vi "CodeBlockSegment.vi"(3 "error in (no error)":errorcluster caption="错误输入（无错误）", 4 "crc_data":dbl[](array[numeric]), 5 "appended path":path) -> (0 "error out":errorcluster caption="错误输出", 1 "Array":dbl[][](array[numeric]), 2 "Cluster":T1)   [LabVIEW 2015]
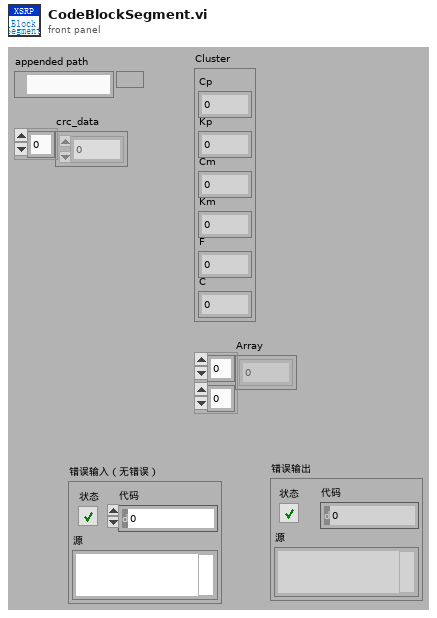
[diagram p1: front panel]
types:
  T1 = cluster{"Cp":dbl, "Kp":dbl, "Cm":dbl, "Km":dbl, "F":dbl, "C":dbl}
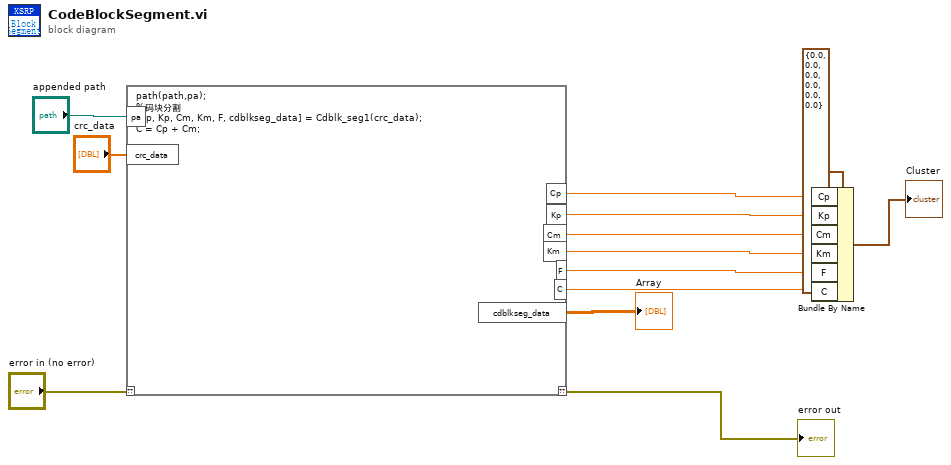
[diagram p0: block diagram]
diagram:
  n1 = script code="path(path,pa);\n%码块分割\n[Cp, Kp, Cm, Km, F, cdblkseg_data] = Cdblk_seg1(crc_data);\nC = Cp + Cm;"("??"="error in (no error)", "pa"="appended path", "crc_data"="crc_data") -> ("??"=→"error out":errorcluster, "Cp"=w10:dbl, "Kp"=w9:dbl, "Cm"=w8:dbl, "Km"=w7:dbl, "F"=w6:dbl, "cdblkseg_data"=→"Array":dbl[][], "C"=w13:dbl)
  n2 = Bundle By Name(cluster=T1 {"Cp"=0.0, "Kp"=0.0, "Cm"=0.0, "Km"=0.0, "F"=0.0, "C"=0.0}, "Cp"=w10, "Kp"=w9, "Cm"=w8, "Km"=w7, "F"=w6, "C"=w13) -> (→"Cluster":T1)
